vi "Convert Decimal Degrees to dms.vi"(1 "Decimal Degrees":dbl=-7.783851 format="%.10f") -> (0 "Deg:Min:Sec":string="-7:47:1.864")   [LabVIEW 2015]
panel:
  out "hours":dbl=0.5189234 format="%.2f"
  out "seconds":dbl=1.863600000001071 format="%.3f"
  out "minutes":dbl=47.0 format="%.2f"
  out "degrees":dbl=-7.0 format="%.2f"
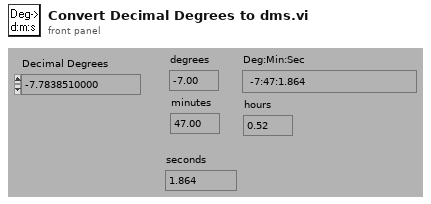
[diagram p1: front panel]
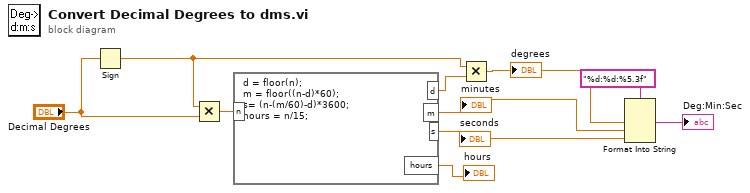
[diagram p0: block diagram]
diagram:
  n1 = Sign(1:"Decimal Degrees") -> (0:w1:dbl)
  n2 = Multiply(x=w1, y="Decimal Degrees") -> (x*y=w4:dbl)
  n3 = formula code="d = floor(n);\nm = floor((n-d)*60);\ns= (n-(m/60)-d)*3600;\nhours = n/15;"("n"=w4) -> ("d"=w2:dbl, "m"=w9:dbl, "s"=w8:dbl, "hours"=→"hours":dbl)
  "minutes" <- w9
  "seconds" <- w8
  n4 = Multiply(x=w1, y=w2) -> (x*y=w3:dbl)
  "degrees" <- w3
  n5 = Format Into String(format string="%d:%d:%5.3f" ("Format String"), w3, w9, w8) -> (resulting string=→"Deg:Min:Sec":string)  [unwired: 2 in, 1 out]
